vi "CarWashTest.vi"(0 "VI Reference In":refnum<vi>, 2 "Label":string, 5 "Wash Option":string, 7 "Car Position":u8=1, 9 "Elapsed Time":dbl=5.0, 11 "error in":errorcluster) -> (4 "VI Reference Out":refnum<vi>, 15 "error out":errorcluster)   [LabVIEW 2016]
uses:
  main/apis/Stimulus/ValueSignal/ValueSignalByPathString.vi
  main/apis/Assert/AssertControlValue/True.vi
  main/apis/Assert/AssertControlValue/Equal.vi
  main/apis/Assert/AssertControlValue/AlmostEqual.vi
  <vilib>/addons/_JKI Toolkits/Caraya/classes/Test/Test.lvclass
  main/apis/Assert/AssertControlValue/AssertControlValue.lvlib
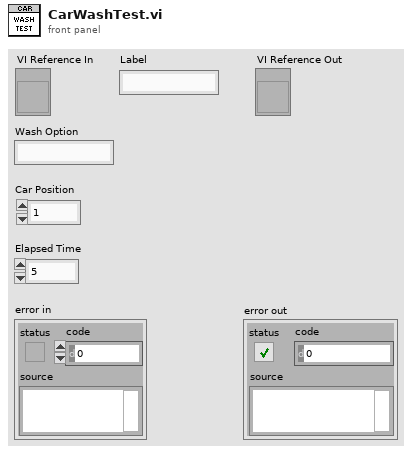
[diagram p1: front panel]
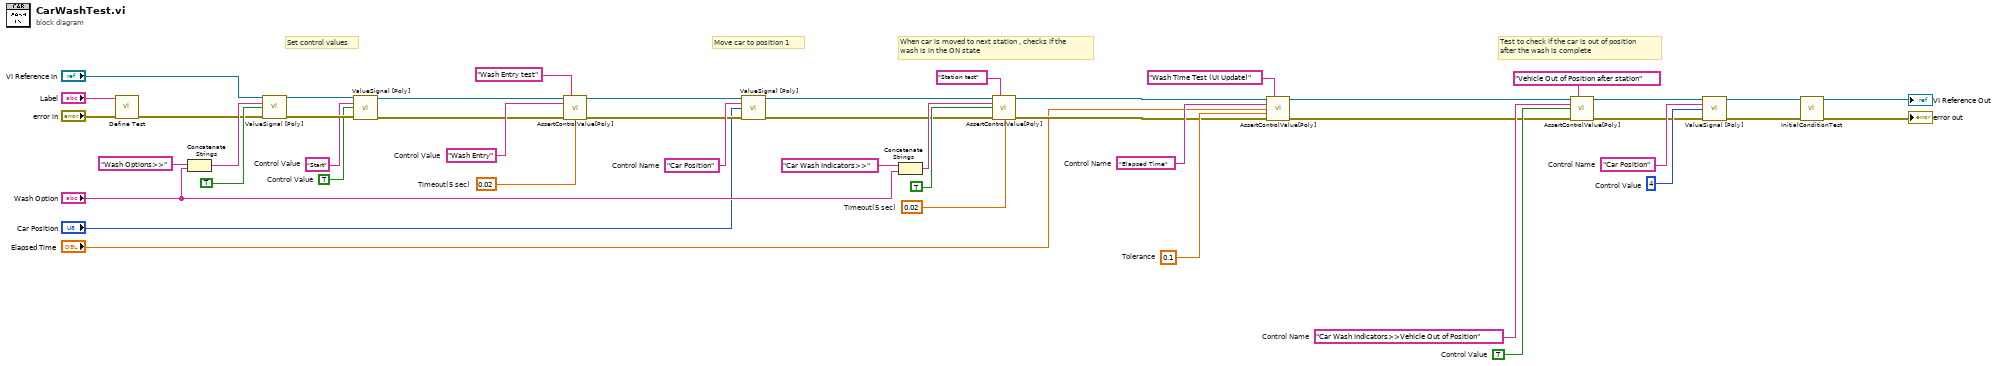
[diagram p0: block diagram]
diagram:
  w15 = "Start"  # Control Value
  w16 = TRUE  # Control Value
  w28 = u8 4  # Control Value
  w29 = "Car Position"  # Control Name
  w34 = TRUE  # Control Value
  w41 = 0.02  # Timeout(5 sec)
  w38 = 0.1  # Tolerance
  w39 = "Elapsed Time"  # Control Name
  w35 = "Car Wash Indicators>>Vehicle Out of Position"  # Control Name
  w45 = "Car Position"  # Control Name
  w46 = 0.02  # Timeout(5 sec)
  w47 = "Wash Entry"  # Control Value
  # "Set control values"
  # "Test to check if the car is out of position \nafter the wash is complete"
  # "When car is moved to next station , checks if the\nwash is in the ON state"
  # "Move car to position 1"
  n1 = call <vilib>:"Define Test.vi"("error in (no error)"="error in", "Label (VI Title)"="Label") -> ("error out"=w9:errorcluster)  [unwired: 9 in]
  n2 = Concatenate Strings("Wash Options>>", "Wash Option") -> (w24:string)
  n3 = call-poly "ValueSignal [Poly].vi"("VI Reference In"="VI Reference In", "Control Name"=w24, "Value (Signaling)"=TRUE, "error in"=w9) -> ("VI Reference Out"=w19:refnum<vi>, "error out"=w21:errorcluster)  [unwired: 10 in]
  n4 = call-poly "ValueSignal [Poly].vi"("VI Reference In"=w19, "Control Name"=w15, "Value (Signaling)"=w16, "error in"=w21) -> ("VI Reference Out"=w17:refnum<vi>, "error out"=w20:errorcluster)  [unwired: 10 in]
  n5 = call-poly "AssertControlValue[Poly].vi"("VI Reference In"=w17, "Label"="Wash Entry test", "Control Name"=w47, "Error In"=w20, "Timeout(5 sec)"=w46) -> ("VI Reference Out"=w43:refnum<vi>, "Error Out"=w44:errorcluster)  [unwired: 9 in]
  n6 = call-poly "ValueSignal [Poly].vi"("VI Reference In"=w43, "Control Name"=w45, "Value (Signaling)"="Car Position", "error in"=w44) -> ("VI Reference Out"=w30:refnum<vi>, "error out"=w6:errorcluster)  [unwired: 10 in]
  n7 = Concatenate Strings("Car Wash Indicators>>", "Wash Option") -> (w13:string)
  n8 = call-poly "AssertControlValue[Poly].vi"("VI Reference In"=w30, "Label"="Station test", "Control Name"=w13, "Control Value"=TRUE, "Error In"=w6, "Timeout(5 sec)"=w41) -> ("VI Reference Out"=w37:refnum<vi>, "Error Out"=w7:errorcluster)  [unwired: 8 in]
  n9 = call-poly "AssertControlValue[Poly].vi"("VI Reference In"=w37, "Label"="Wash Time Test (UI Update)", "Control Name"=w39, "Control Value"="Elapsed Time", "Tolerance"=w38, "Error In"=w7) -> ("VI Reference Out"=w31:refnum<vi>, "Error Out"=w32:errorcluster)  [unwired: 8 in]
  n10 = call-poly "AssertControlValue[Poly].vi"("VI Reference In"=w31, "Label"="Vehicle Out of Position after station", "Control Name"=w35, "Control Value"=w34, "Error In"=w32) -> ("VI Reference Out"=w27:refnum<vi>, "Error Out"=w26:errorcluster)  [unwired: 9 in]
  n11 = call-poly "ValueSignal [Poly].vi"("VI Reference In"=w27, "Control Name"=w29, "Value (Signaling)"=w28, "error in"=w26) -> ("VI Reference Out"=w2:refnum<vi>, "error out"=w4:errorcluster)  [unwired: 10 in]
  n12 = call "InitialConditionTest.vi"("VI Reference In"=w2, "error in"=w4) -> ("VI Reference Out"=→"VI Reference Out":refnum<vi>, "error out"=→"error out":errorcluster)  [unwired: 12 in]
